vi "medicaoIXV.vi"() -> ()   [LabVIEW 2012]
uses:
  <vilib>/Utility/file.llb/Write To Spreadsheet File (string).vi
  <vilib>/Utility/file.llb/Write To Spreadsheet File (DBL).vi
  <instrlib>/Agilent 6XXX Series/Agilent 6XXX Series.lvlib
panel:
  out "stop2":bool
  out "reset graph":bool=TRUE
  out "array":dbl[][](array[numeric])
  in  "Tab Control":enum32{"Entrada de dados", "Saída de dados"}(tab)
  out "ON/OFF":bool
  in  "Pontos":dbl
  in  "Tensão máxima":dbl
  in  "Nome da célula":string
  in  "Local":path
  in  "Delay(ms)":dbl
  in  "Start":bool
  in  "Print Screen":bool
  out "IXV":cluster{"Y":dbl[], "Y":dbl[]}[](graph)
  out "output voltage":dbl
  out "Tensao Atual":dbl
  out "Corrente Atual":dbl
  out "Ponto Atual":i32
  out "TABELA DE DADOS\nTensão(fonte)     Tensão                  Corrente            Pontos":dbl[][](array[numeric]) caption="all rows" format="%0.3f"
  in  "stop":bool
  out "ON/OFF":bool
  in  "CorrenteGraph":dbl
  in  "error in (no error)":errorcluster
  out "error out":errorcluster
  in  "TensaoGraph":dbl
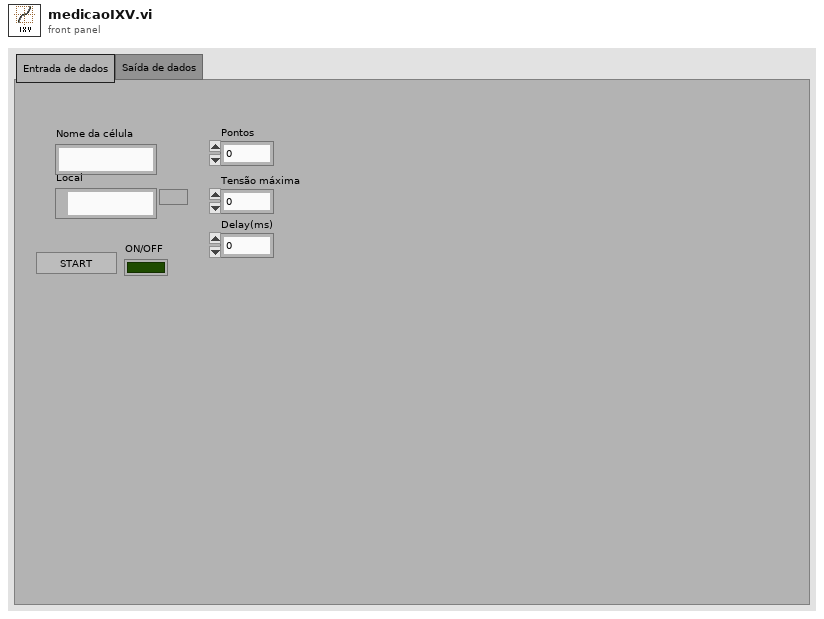
[diagram p1: front panel]
types:
  T1 = typedef "imagedata.ctl" = cluster{"image type":i32, "image depth":i32, "image":u8[], "mask":u8[], "colors":u32[], "Rectangle":cluster{"left":i16, "top":i16, "right":i16, "bottom":i16}}
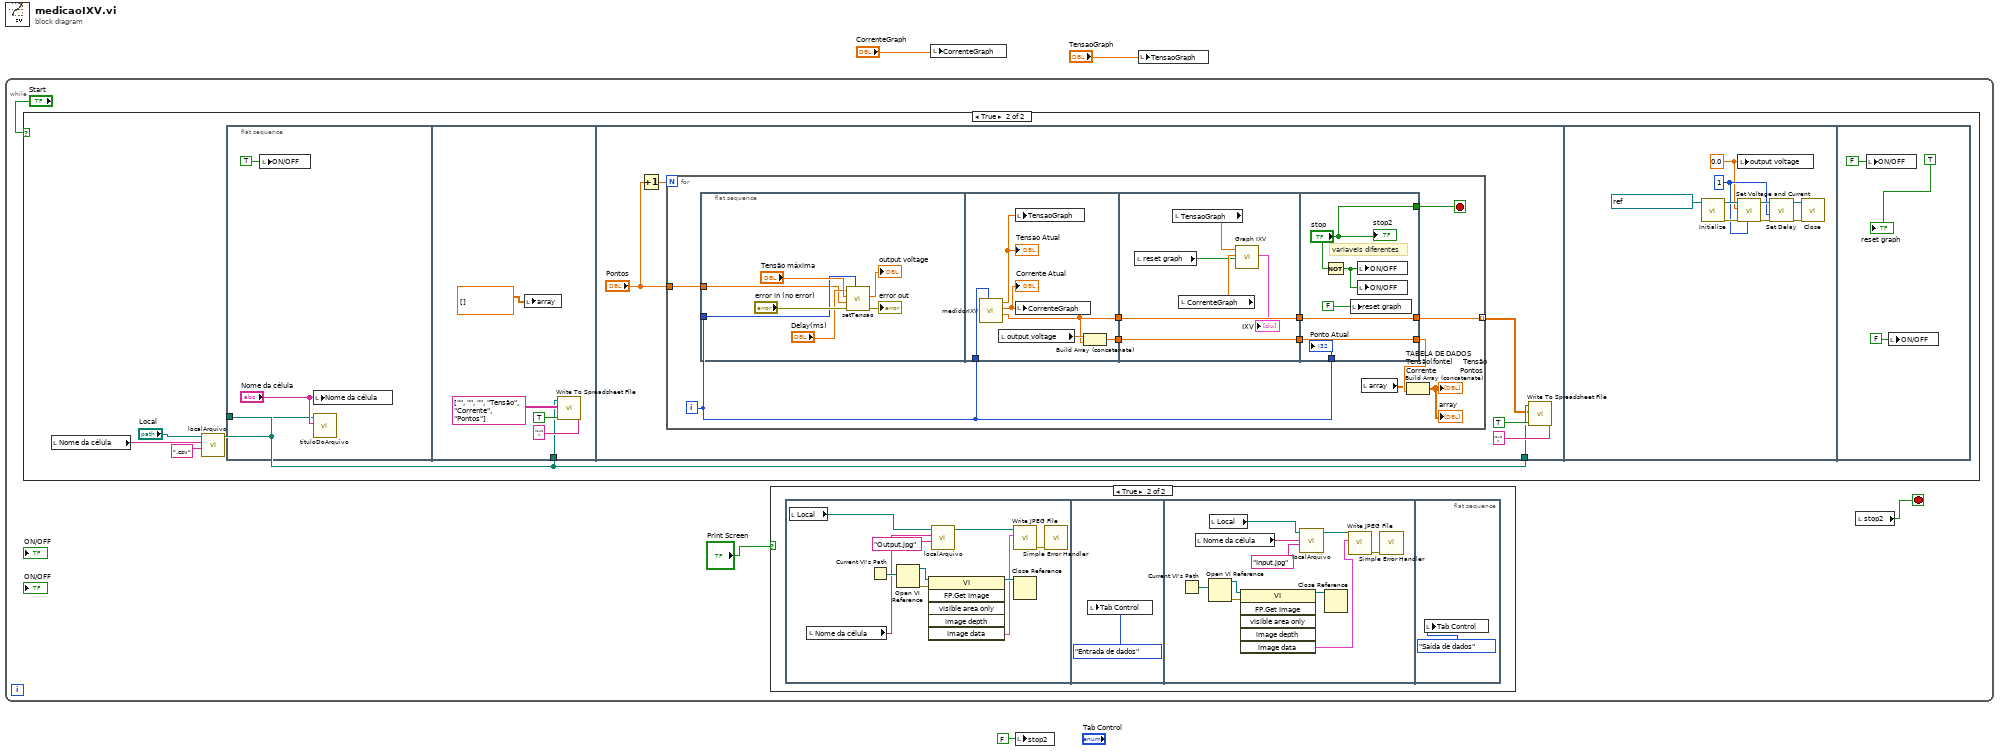
[diagram p0: block diagram]
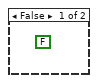
[diagram p3: hidden frame]
diagram:
  n1 = while {
    stop <- w4 stop-if-true
    n2 = case shown="True" "Start" {
      frame False {
        (unwired) FALSE
      }
      frame True {
        n3 = local read "Nome da célula"() -> (w30:string)
        n4 = call "localArquivo.vi"("extensão"=".csv", "Nome do arquivo"=w30, "Local"="Local") -> ("Path"=w29:path)  [unwired: 8 in]
        n5 = flat-sequence {
          tunnel: w29 -> [w34]
          tunnel: w29 -> [w37]
          tunnel: w29 -> [w44]
          frame #0 {
            n6 = local write "ON/OFF"(TRUE ("ON/OFF")) -> ()
            n7 = local write "Nome da célula"("Nome da célula") -> ()
            n8 = call "tituloDoArquivo.vi"("Nome da célula"="Nome da célula", "file path (dialog if empty)"=w34) -> ()  [unwired: 10 in]
          }
          frame #1 {
            n9 = local write "array"(dbl[][] [] ("array")) -> ()
            n10 = call-poly <vilib>:"Write To Spreadsheet File.vi"("delimiter (\\t)"=";" ("delimiter (\\t)"), "append to file? (new file:F)"=TRUE, "2D data"=string[][] [["", "", ""], ["Tensão", "Corrente", "Pontos"]], "file path (dialog if empty)"=w37) -> ()  [unwired: 4 in, 1 out]
          }
          frame #2 {
            n11 = Increment(x="Pontos") -> (x+1=w43:dbl)
            n12 = for {
              N: w43 -> [_]
              tunnel: [w56] -> w41 mode=indexing
              tunnel: "Pontos" -> [w57]
              i -> [w48]
              stop <- w47 stop-if-true
              n13 = flat-sequence {
                tunnel: w57 -> [w60]
                tunnel: w48 -> [w61]
                tunnel: w48 -> [w70]
                tunnel: [w65] -> w55
                tunnel: [w67] -> w54
                tunnel: w55 -> [w76]
                tunnel: w54 -> [w75]
                tunnel: [w76] -> w50
                tunnel: [w75] -> w49
                tunnel: [w81] -> w53
                tunnel: [w82] -> w56
                tunnel: w50 -> [w82]
                tunnel: w49 -> [w81]
                tunnel: w48 -> [w80]
                tunnel: ["stop"] -> w47
                frame #0 {
                  n14 = call "setTensao.vi"("Ponto"=w61, "error in (no error)"="error in (no error)", "Pontos"=w60, "Tensão máxima"="Tensão máxima", "delay(ms)"="Delay(ms)") -> ("error out"=→"error out":errorcluster, "output voltage"=→"output voltage":dbl)  [unwired: 5 in]
                }
                frame #1 {
                  n15 = call "medidorIXV.vi"("Ponto"=w70) -> ("Array"=w65:dbl[], "Corrente Atual"=w69:dbl, "Tensao Atual"=w68:dbl)  [unwired: 8 in]
                  "Corrente Atual" <- w69
                  "Tensao Atual" <- w68
                  n16 = local read "output voltage"() -> (w66:dbl)
                  n17 = local write "TensaoGraph"(w68) -> ()
                  n18 = local write "CorrenteGraph"(w69) -> ()
                  n19 = Build Array (concatenate)(w66, w65) -> (w67:dbl[])
                }
                frame #2 {
                  n20 = local read "reset graph"() -> (w71:bool)
                  n21 = local read "TensaoGraph"() -> (w74:dbl)
                  n22 = local read "CorrenteGraph"() -> (w73:dbl)
                  n23 = call "Graph IXV"("Reset"=w71, "Y Input"=w73, "X Input"=w74) -> ("XY Graph"=→"IXV":cluster{"Y":dbl[], "Y":dbl[]}[])  [unwired: 2 in, 6 out]
                }
                frame #3 {
                  # "variaveis diferentes"
                  n24 = Not(x="stop") -> (.not. x?=w77:bool)
                  n25 = local write "reset graph"(FALSE) -> ()
                  n26 = local write "ON/OFF"(w77) -> ()
                  n27 = local write "ON/OFF"(w77) -> ()
                  "Ponto Atual" <- w80
                  "stop2" <- "stop"
                }
              }
              n28 = local read "array"() -> (w52:dbl[][])
              n29 = Build Array (concatenate)(w52, w53) -> (→"TABELA DE DADOS\nTensão(fonte)     Tensão                  Corrente            Pontos" →"array":dbl[][])
            }
            n30 = call-poly <vilib>:"Write To Spreadsheet File.vi"("delimiter (\\t)"=";" ("delimiter (\\t)"), "append to file? (new file:F)"=TRUE, "2D data"=w41, "file path (dialog if empty)"=w44) -> ()  [unwired: 4 in, 1 out]
          }
          frame #3 {
            w83 = 0.0 ("voltage (0 V)")
            w86 = u8 1 ("channel (1)")
            n31 = call <instrlib>:"Initialize.vi"("VISA resource name"=refnum<visa-resource-name> "GPIB0::5::INSTR") -> ("error out"=w88:errorcluster, "VISA resource name out"=w87:refnum<visa-resource-name>)  [unwired: 9 in]
            n32 = local write "output voltage"(w83) -> ()
            n33 = call <instrlib>:"Set Voltage and Current.vi"("channel (1)"=w86, "error in (no error)"=w88, "voltage (0 V)"=w83, "VISA resource name"=w87) -> ("error out"=w89:errorcluster, "VISA resource name out"=w90:refnum<visa-resource-name>)  [unwired: 6 in]
            n34 = call <instrlib>:"Set Delay.vi"("error in (no error)"=w89, "channel (1)"=w86, "VISA resource name"=w90) -> ("error out"=w84:errorcluster, "VISA resource name out"=w85:refnum<visa-resource-name>)  [unwired: 7 in]
            n35 = call <instrlib>:"Close.vi"("error in (no error)"=w84, "VISA resource name"=w85) -> ()  [unwired: 9 in, 1 out]
          }
          frame #4 {
            n36 = local write "ON/OFF"(FALSE) -> ()
            n37 = local write "ON/OFF"(FALSE ("ON/OFF")) -> ()
            "reset graph" <- TRUE
          }
        }
      }
    }
    n38 = case shown="True" "Print Screen" {
      frame False {
      }
      frame True {
        n39 = flat-sequence {
          frame #0 {
            n40 = local read "Local"() -> (w8:path)
            n41 = local read "Nome da célula"() -> (w7:string)
            n42 = Current VI's Path() -> (path=w13:path)
            n43 = Open VI Reference(vi path=w13) -> (vi reference=w14:refnum<vi>, error out=w15:errorcluster)  [unwired: 5 in]
            n44 = invoke class="VI" method="FP.Get Image"(reference=w14, error in=w15) -> (reference out=w12:refnum<vi>, "image data"=w11:T1)  [unwired: 4 in, 4 out]
            n45 = call "localArquivo.vi"("extensão"="Output.jpg", "Nome do arquivo"=w7, "Local"=w8) -> ("Path"=w16:path)  [unwired: 8 in]
            n46 = call <vilib>:"Write JPEG File.vi"("image data"=w11, "path to JPEG file"=w16) -> ("error out"=w10:errorcluster)  [unwired: 8 in, 1 out]
            n47 = Close Reference(reference=w12) -> ()  [unwired: 1 in, 1 out]
            n48 = call <vilib>:"Simple Error Handler.vi"("error in (no error)"=w10) -> ()  [unwired: 4 in, 5 out]
          }
          frame #1 {
            n49 = local write "Tab Control"(enum32{"Entrada de dados", "Saída de dados"}."Entrada de dados" ("Tab Control")) -> ()
          }
          frame #2 {
            n50 = Current VI's Path() -> (path=w26:path)
            n51 = local read "Nome da célula"() -> (w19:string)
            n52 = Open VI Reference(vi path=w26) -> (vi reference=w25:refnum<vi>, error out=w24:errorcluster)  [unwired: 5 in]
            n53 = local read "Local"() -> (w18:path)
            n54 = invoke class="VI" method="FP.Get Image"(reference=w25, error in=w24) -> (reference out=w27:refnum<vi>, "image data"=w22:T1)  [unwired: 4 in, 4 out]
            n55 = call "localArquivo.vi"("extensão"="Input.jpg", "Nome do arquivo"=w19, "Local"=w18) -> ("Path"=w21:path)  [unwired: 8 in]
            n56 = Close Reference(reference=w27) -> ()  [unwired: 1 in, 1 out]
            n57 = call <vilib>:"Write JPEG File.vi"("image data"=w22, "path to JPEG file"=w21) -> ("error out"=w23:errorcluster)  [unwired: 8 in, 1 out]
            n58 = call <vilib>:"Simple Error Handler.vi"("error in (no error)"=w23) -> ()  [unwired: 4 in, 5 out]
          }
          frame #3 {
            n59 = local write "Tab Control"(enum32{"Entrada de dados", "Saída de dados"}."Saída de dados" ("Tab Control")) -> ()
          }
        }
      }
    }
    n60 = local read "stop2"() -> (w4:bool)
  }
  n61 = local write "CorrenteGraph"("CorrenteGraph") -> ()
  n62 = local write "stop2"(FALSE ("stop2")) -> ()
  n63 = local write "TensaoGraph"("TensaoGraph") -> ()
